vi "Intake IR.vi"(7 "Unload?":bool, 11 "Speed":dbl) -> (3 "Speeeeeeed":dbl)   [LabVIEW 2015]
uses:
  Common Code/Intake Commands Cluster.ctl
  Common Code/Intake Commands.ctl
  Common Code/Intake Mode.ctl
panel:
  in  "Intake Commands Cluster":T1={"Intake Commands"=enum."Load", "Intake Mode"=enum."Auto", "Override IR"=FALSE}
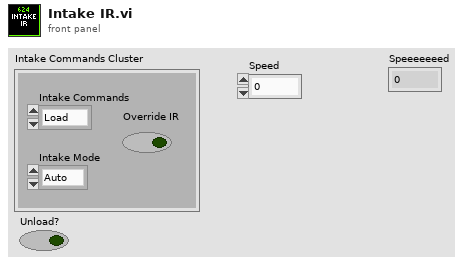
[diagram p1: front panel]
types:
  T1 = typedef "Intake Commands Cluster.ctl" = cluster{"Intake Commands":T2, "Intake Mode":T3, "Override IR":bool}
  T2 = typedef "Intake Commands.ctl" = enum16{"Unload", "Load", "Pull up", "Drop low", "Idle", "Lift Half"}
  T3 = typedef "Intake Mode.ctl" = enum16{"Safe", "Auto", "Manual"}
  T4 = typedef "WPI_DigitalInputDevRef.ctl" = cluster{"DevStatus":errorcluster, "DIO Channel":T5}
  T5 = typedef "FPGA_DIOChannel.ctl" = enum8{"DIO 0", "DIO 1", "DIO 2", "DIO 3", "DIO 4", "DIO 5", "DIO 6", "DIO 7", "DIO 8", "DIO 9", "DIO MXP 0", "DIO MXP 1", "DIO MXP 2", "DIO MXP 3", "DIO MXP 4", "DIO MXP 5", "DIO MXP 6", "DIO MXP 7", "DIO MXP 8", "DIO MXP 9", "DIO MXP 10", "DIO MXP 11", "DIO MXP 12", "DIO MXP 13", "DIO MXP 14", "DIO MXP 15", "Invalid"}
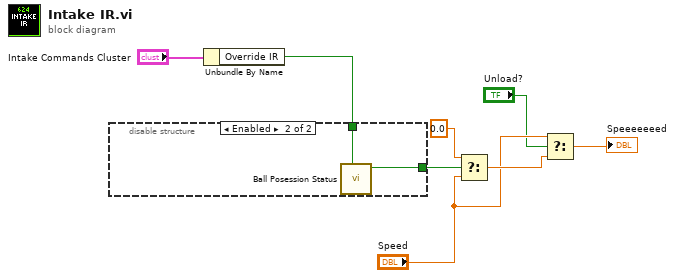
[diagram p0: block diagram]
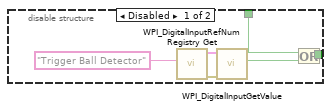
[diagram p2: hidden frame]
diagram:
  n1 = Unbundle By Name("Intake Commands Cluster") -> ("Override IR"=w6:bool)
  n2 = disable-structure shown="Enabled" {
    disable-tunnel: [w14 w15] -> w7
    disable-tunnel: w6 -> [w12 w16]
    frame Disabled {
      n3 = call <vilib>:"WPI_DigitalInputRefNum Registry Get.vi"("refnum name"="Trigger Ball Detector") -> ("error out"=w11:errorcluster, "DigitalInputDevRef"=w10:T4)  [unwired: 9 in]
      n4 = call <vilib>:"WPI_DigitalInputGetValue.vi"("error in (no error)"=w11, "DigitalInputDevRef"=w10) -> ("Value"=w13:bool)  [unwired: 7 in, 2 out]
      n5 = Or(x=w12, y=w13) -> (x .or. y?=w14:bool)
    }
    frame Enabled {
      n6 = call "Ball Posession Status.vi"("Override to True?"=w16) -> ("Ball Posessed?"=w15:bool)  [unwired: 10 in]
    }
  }
  n7 = Select(t=0.0, s=w7, f="Speed") -> (s? t:f=w4:dbl)
  n8 = Select(t="Speed", s="Unload?", f=w4) -> (s? t:f=→"Speeeeeeed":dbl)
